vi "Trigger Video (SubVI).vi"(6 "Sync":u16(ring) items=["Field", "Line", "Odd", "Even", "LineNum"], 7 "Lines":dbl(knob) scale=0.0..525.0, 8 "Standard":u16(ring) items=["NTSC", "PAL"], 9 "Polarity":u16(ring) items=["Inverted", "Normal"], 10 "Canal":u16(ring) items=["Canal 1", "Canal 2"], 11 "String de Entrada":string) -> (2 "String de Salida":string, 3 "String de Tipo":string)   [LabVIEW 2014]
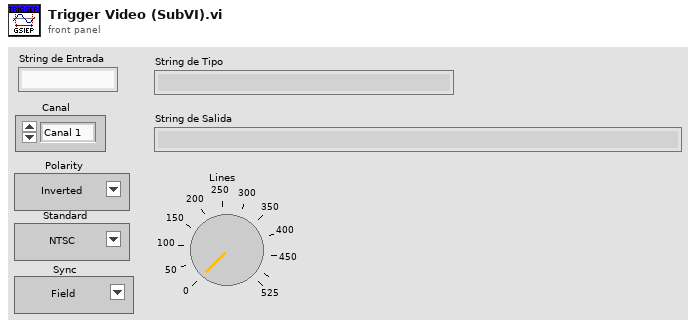
[diagram p1: front panel]
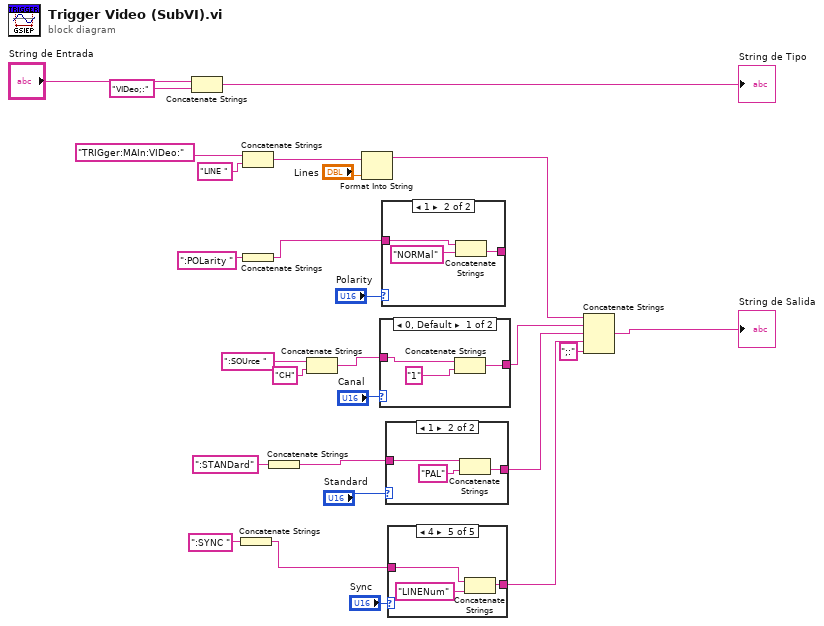
[diagram p0: block diagram]
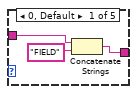
[diagram p2: hidden frame]
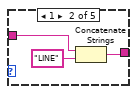
[diagram p3: hidden frame]
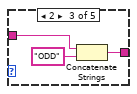
[diagram p4: hidden frame]
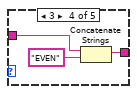
[diagram p5: hidden frame]
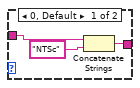
[diagram p6: hidden frame]
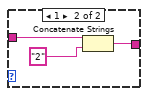
[diagram p7: hidden frame]
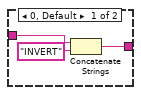
[diagram p8: hidden frame]
diagram:
  n1 = Concatenate Strings("String de Entrada", "VIDeo;:") -> (→"String de Tipo":string)
  n2 = Concatenate Strings(":SYNC ") -> (w18:string)
  n3 = Concatenate Strings("TRIGger:MAIn:VIDeo:", "LINE ") -> (w5:string)
  n4 = Concatenate Strings(":POLarity ") -> (w8:string)
  n5 = Concatenate Strings(":STANDard") -> (w15:string)
  n6 = Concatenate Strings(":SOUrce ", "CH") -> (w11:string)
  n7 = Format Into String(initial string=w5, "Lines") -> (resulting string=w21:string)  [unwired: 2 in, 1 out]
  n8 = case shown="0, Default" "Canal" {
    tunnel: w11 -> [w28 w31]
    tunnel: [w27 w30] -> w22
    frame 0, Default {
      n9 = Concatenate Strings(w28, "1") -> (w27:string)
    }
    frame 1 {
      n10 = Concatenate Strings(w31, "2") -> (w30:string)
    }
  }
  n11 = case shown="1" "Polarity" {
    tunnel: w8 -> [w34 w37]
    tunnel: [w33 w36] -> _
    frame 0, Default {
      n12 = Concatenate Strings(w34, "INVERT") -> (w33:string)
    }
    frame 1 {
      n13 = Concatenate Strings(w37, "NORMal") -> (w36:string)
    }
  }
  n14 = case shown="1" "Standard" {
    tunnel: w15 -> [w41 w44]
    tunnel: [w39 w42] -> w23
    frame 0, Default {
      n15 = Concatenate Strings(w41, "NTSc") -> (w39:string)
    }
    frame 1 {
      n16 = Concatenate Strings(w44, "PAL") -> (w42:string)
    }
  }
  n17 = case shown="4" "Sync" {
    tunnel: w18 -> [w46 w49 w52 w55 w58]
    tunnel: [w45 w48 w51 w54 w57] -> w24
    frame 0, Default {
      n18 = Concatenate Strings(w46, "FIELD") -> (w45:string)
    }
    frame 1 {
      n19 = Concatenate Strings(w49, "LINE") -> (w48:string)
    }
    frame 2 {
      n20 = Concatenate Strings(w52, "ODD") -> (w51:string)
    }
    frame 3 {
      n21 = Concatenate Strings(w55, "EVEN") -> (w54:string)
    }
    frame 4 {
      n22 = Concatenate Strings(w58, "LINENum") -> (w57:string)
    }
  }
  n23 = Concatenate Strings(w21, w22, w23, w24, ";:") -> (→"String de Salida":string)
